vi "niScope EX Getting Started.vi"() -> ()   [LabVIEW 2021]
doc: "Example: Getting Started\n\nRecommended Input Signal: 100 kHz, 1.8 Vpp, sine wave\n\nDevices Supported: Refer to NI Example Finder\n\nLabVIEW Description:\n\nThis example opens a session to the NI-SCOPE driver by passing in the device's resource name to the Initialize VI. The resource name is a unique identifier for your National Instruments' hardware product. It can be found (and changed) by running Measurement & Automation Explorer (MAX). A shortcut to MAX is placed on your desktop when NI-SCOPE or NI-DAQ is installed.\n\nThe session handle returned from the Initialize VI is a parameter to all VIs in the NI-SCOPE driver. Only one session may be opened at a time for your oscilloscope, and every session should be closed by calling the Close vi. The session should be closed even when an error occurs.\n\nThe Auto Setup VI takes several acquisitions to measure the amplitude and frequency of the input signal. This allows it to optimally set properties such as the sample rate, vertical range, and minimum record length. The Read VI, initiates an acquisition, waits for it to finish, and fetches the data from the oscilloscope. The data is returned as a bundle of the initial x, x increment, and waveform. Initial x is the time of the first point in the waveform relative to the trigger, while the x increment is the time between two points in the waveform. This bundle may be directly wired to a waveform graph, to display the waveform with timing information. \n\nThe Error Handler VI translates any error messages into text messages."
uses:
  <instrlib>/niScope/Acquire/niScope Multi Read Cluster.vi
panel:
  in  "Simulate?":bool
  out "Waveform Graph":T1(graph)
  in  "resource name":refnum<k15>="Dev1" caption="Resource Name(s)"
  in  "Channel(s)":string="0"
  # "Overview: Demonstrates the minimal code needed to use NI-SCOPE.\nRequirements: NI-SCOPE\nInstructions: \n1.  Select the appropriate device in the Resource Name control.\n2.  Enter the channels you would like to acquire from in the Channel(s) control.\n3.  Run the VI."
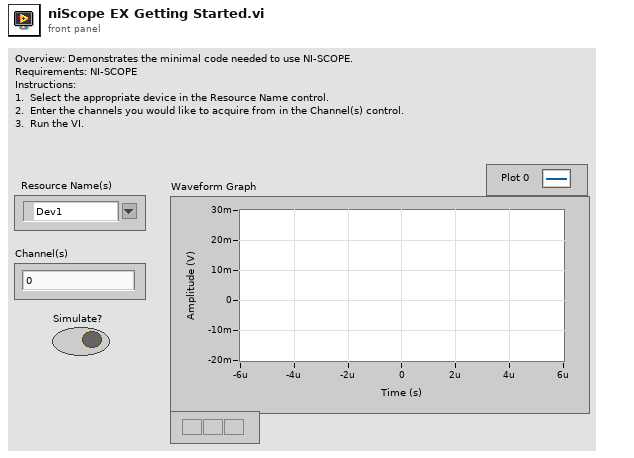
[diagram p1: front panel]
types:
  T1 = cluster{"relativeInitialX":dbl, "xIncrement":dbl, "wfm":dbl[]}[]
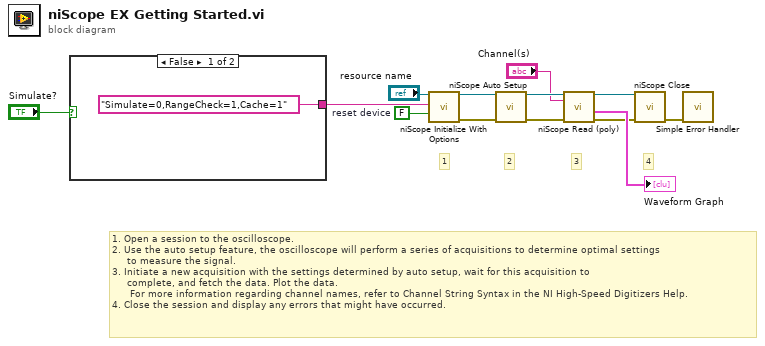
[diagram p0: block diagram]
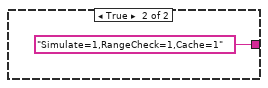
[diagram p2: hidden frame]
diagram:
  w10 = FALSE  # reset device
  # "1. Open a session to the oscilloscope.\n2. Use the auto setup feature, the oscilloscope will perform a series of acquisitions to determine optimal settings\n     to measure the signal.\n3. Initiate a new acquisition with the settings determined by auto setup, wait for this acquisition to\n     complete, and fetch the data. Plot the data.\n      For more information regarding channel names, refer to Channel String Syntax in the NI High-Speed Digitizers Help.\n4. Close the session and display any errors that might have occurred."
  # "4"
  # "3"
  # "2"
  # "1"
  n1 = case shown="False" "Simulate?" {
    tunnel: ["Simulate=0,RangeCheck=1,Cache=1" ("option string") "Simulate=1,RangeCheck=1,Cache=1" ("option string")] -> w1
    frame False {
    }
    frame True {
    }
  }
  n2 = call <instrlib>:"niScope Initialize With Options.vi"("resource name"="resource name", "option string"=w1, "reset device"=w10) -> ("instrument handle"=w13:refnum<k15>, "error out"=w12:errorcluster)  [unwired: 11 in]
  n3 = call <instrlib>:"niScope Auto Setup.vi"("instrument handle"=w13, "error in"=w12) -> ("instrument handle out"=w9:refnum<k15>, "error out"=w8:errorcluster)  [unwired: 12 in]
  n4 = call-poly <instrlib>:"niScope Read (poly).vi"("error in"=w8, "channels"="Channel(s)", "instrument handle"=w9) -> ("error out"=w5:errorcluster, "waveform"=→"Waveform Graph":T1, "instrument handle out"=w4:refnum<k15>)  [unwired: 5 in, 1 out]
  n5 = call <instrlib>:"niScope Close.vi"("instrument handle"=w4, "error in"=w5) -> ("error out"=w3:errorcluster)  [unwired: 13 in]
  n6 = call <vilib>:"Simple Error Handler.vi"("error in (no error)"=w3) -> ()  [unwired: 4 in, 5 out]
